vi "Check Properties Equal.vi"(8 "error in":errorcluster, 9 "Ignore Properties":string[](array[string]), 10 "BaseNodeType 2":refnum<k24>, 11 "BaseNodeType 1":refnum<k24>) -> (0 "error out":errorcluster, 1 "Equal?":bool, 2 "BaseNodeType 2":refnum<k24>, 3 "BaseNodeType 1":refnum<k24>, 4 "Inequality context":string)   [LabVIEW 2017, in "SLSC Switch Import Export Unit Tests.lvclass"]
uses:
  SLSC Switch Import Export Unit Tests.lvclass
  NationalInstruments.VeriStand.SystemStorage
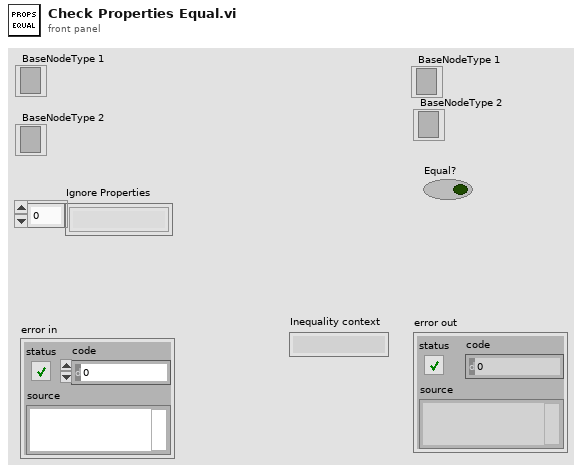
[diagram p1: front panel]
types:
  T1 = cluster{"ForceDownload":bool, "Path":string, "RTDestination":string, "Type":i32, "Version":string}
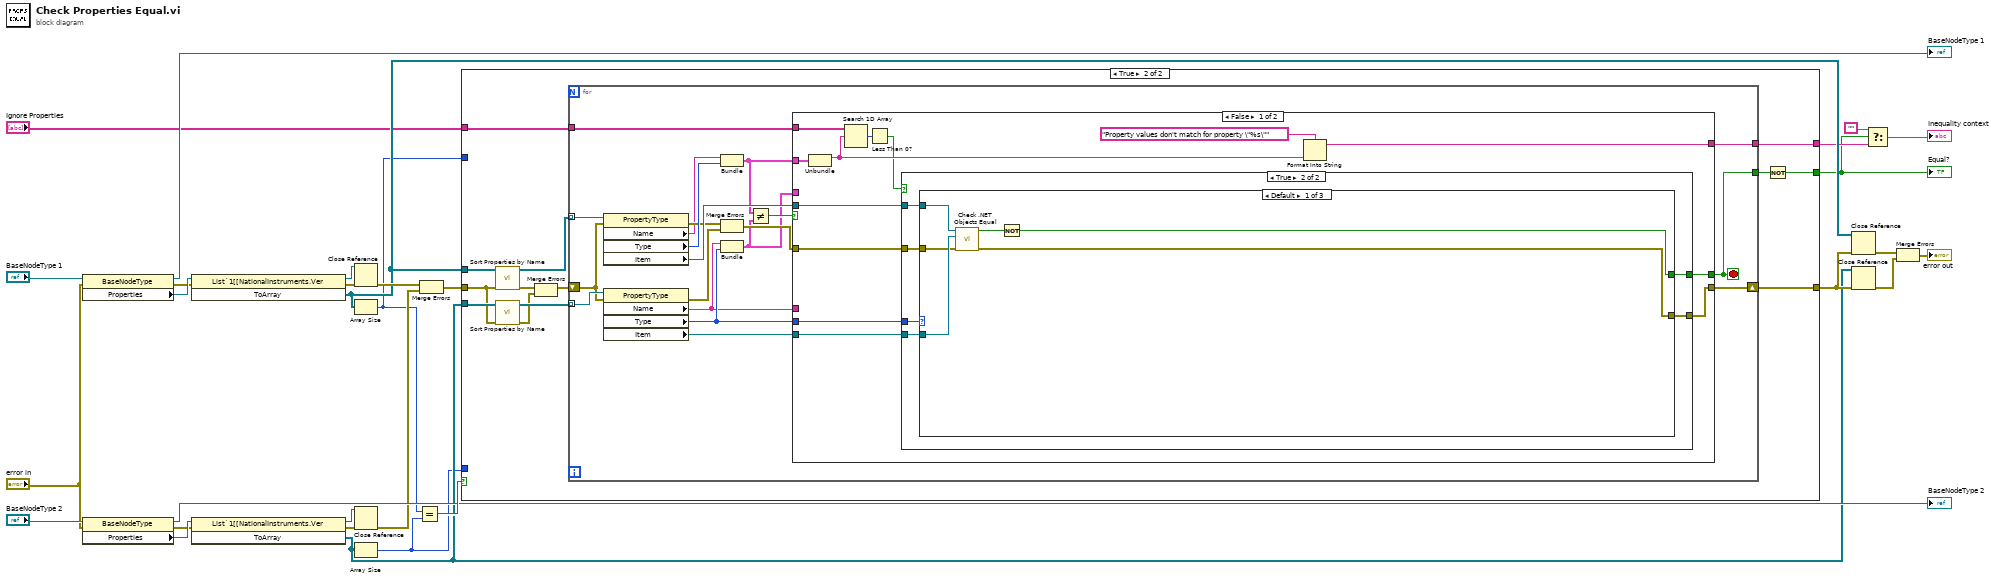
[diagram p0: block diagram]
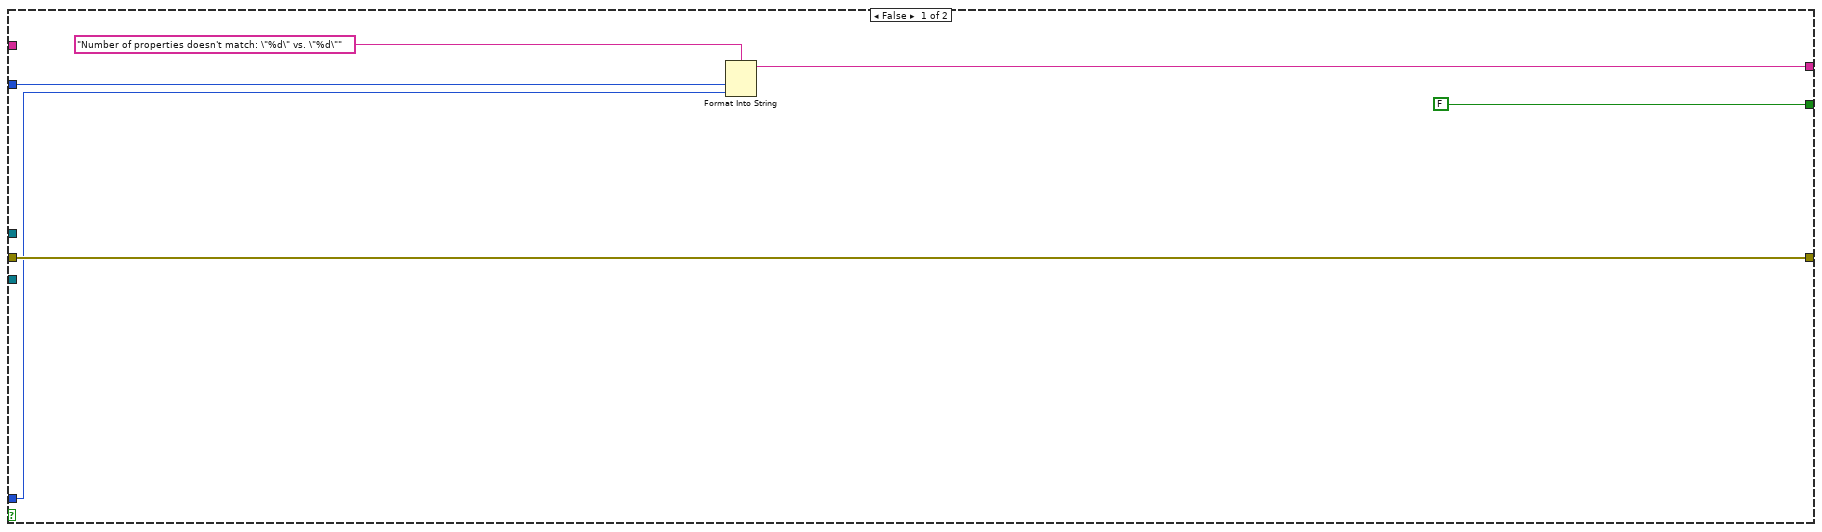
[diagram p2: hidden frame]
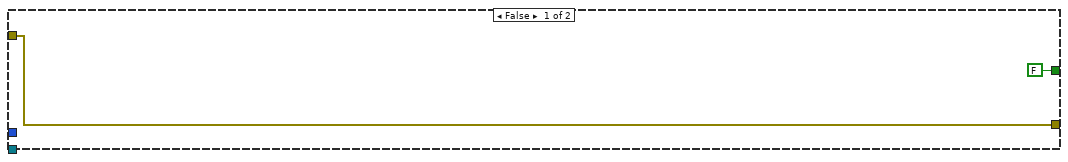
[diagram p3: hidden frame]
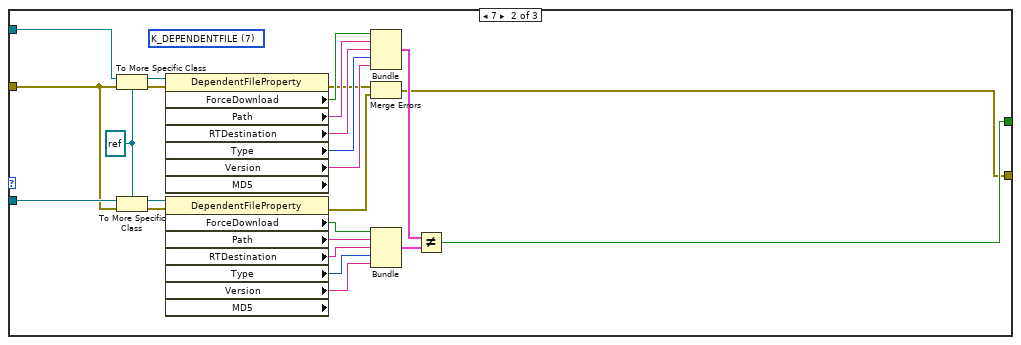
[diagram p4: hidden frame]
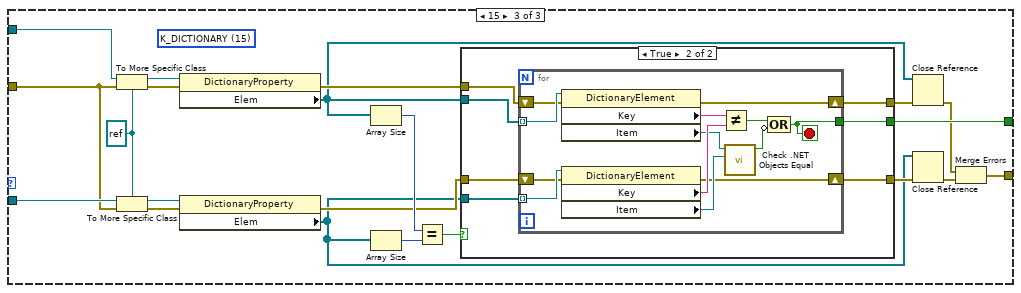
[diagram p5: hidden frame]
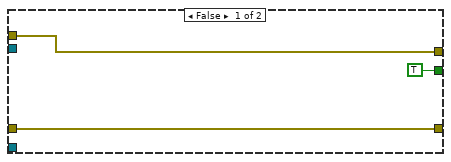
[diagram p6: hidden frame]
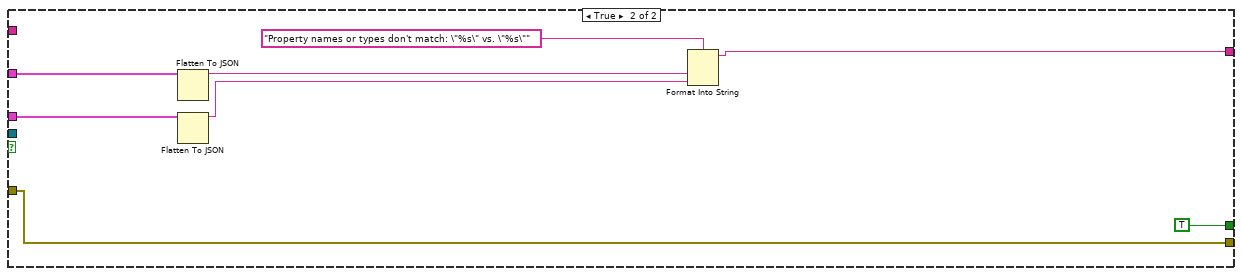
[diagram p7: hidden frame]
diagram:
  n1 = property class="BaseNodeType"(reference="BaseNodeType 1", error in="error in") -> (reference out=→"BaseNodeType 1":refnum<k24>, error out=w22:errorcluster, "Properties"=w29:refnum<k24>)
  n2 = property class="BaseNodeType"(reference="BaseNodeType 2", error in="error in") -> (reference out=→"BaseNodeType 2":refnum<k24>, error out=w21:errorcluster, "Properties"=w27:refnum<k24>)
  n3 = invoke class="List`1[[NationalInstruments.Ver" method="ToArray"(reference=w29, error in=w22) -> (reference out=w19:refnum<k24>, error out=w20:errorcluster, "ToArray"=w12:refnum<k24>[])  [unwired: 1 in]
  n4 = invoke class="List`1[[NationalInstruments.Ver" method="ToArray"(reference=w27, error in=w21) -> (reference out=w17:refnum<k24>, error out=w18:errorcluster, "ToArray"=w11:refnum<k24>[])  [unwired: 1 in]
  n5 = Close Reference(reference=w19, error in (no error)=w20) -> (error out=w16:errorcluster)
  n6 = Array Size(array=w12) -> (size(s)=w7:i32)
  n7 = Close Reference(reference=w17, error in (no error)=w18) -> (error out=w15:errorcluster)
  n8 = Array Size(array=w11) -> (size(s)=w6:i32)
  n9 = Equal?(x=w7, y=w6) -> (x = y?=w25:bool)
  n10 = Merge Errors(w16, w15) -> (w14:errorcluster)
  n11 = case shown="True" w25 {
    tunnel: w12 -> [_ w43]
    tunnel: w11 -> [_ w41]
    tunnel: [FALSE w49] -> w3
    tunnel: w14 -> [w35 w39]
    tunnel: [w35 w47] -> w13
    tunnel: w7 -> [w34 _]
    tunnel: w6 -> [w33 _]
    tunnel: [w32 w46] -> w4
    tunnel: "Ignore Properties" -> [_ w45]
    frame False {
      n12 = Format Into String(format string="Number of properties doesn't match: \"%d\" vs. \"%d\"", w34, w33) -> (resulting string=w32:string)  [unwired: 2 in, 1 out]
    }
    frame True {
      n13 = call "Sort Properties by Name.vi"("error in (no error)"=w39, "properties"=w43) -> ("error out"=w44:errorcluster, "sorted properties"=w42:refnum<k24>[])  [unwired: 8 in]
      n14 = call "Sort Properties by Name.vi"("error in (no error)"=w39, "properties"=w41) -> ("error out"=w37:errorcluster, "sorted properties"=w40:refnum<k24>[])  [unwired: 8 in]
      n15 = Merge Errors(w44, w37) -> (w38:errorcluster)
      n16 = for {
        tunnel: w42 -> [w68] mode=indexing
        tunnel: w40 -> [w67] mode=indexing
        tunnel: [w61] -> w48
        shift-right: [w56] -> w47
        shift-left: w38 -> [w60]
        tunnel: [w53] -> w46
        tunnel: w45 -> [w50]
        stop <- w61 stop-if-true
        n17 = property class="PropertyType"(reference=w68, error in=w60) -> (error out=w59:errorcluster, "Name"=w55:string, "Type"=w63:i32, "Item"=w65:refnum<k24>)  [unwired: 1 out]
        n18 = property class="PropertyType"(reference=w67, error in=w60) -> (error out=w58:errorcluster, "Name"=w54:string, "Type"=w64:i32, "Item"=w66:refnum<k24>)  [unwired: 1 out]
        n19 = Bundle("Name"=w55, "Type"=w63) -> (w52:cluster{"Name":string, "Type":i32})  [unwired: 1 in]
        n20 = Merge Errors(w59, w58) -> (w57:errorcluster)
        n21 = Bundle("Name"=w54, "Type"=w64) -> (w51:cluster{"Name":string, "Type":i32})  [unwired: 1 in]
        n22 = Not Equal?(x=w52, y=w51) -> (x != y?=w62:bool)
        n23 = case shown="False" w62 {
          tunnel: w66 -> [w80 _]
          tunnel: w65 -> [w79 _]
          tunnel: w64 -> [w78 _]
          tunnel: [w81 TRUE] -> w61
          tunnel: w57 -> [w77 w170]
          tunnel: [w76 w170] -> w56
          tunnel: w54 -> [_ _]
          tunnel: [w74 w168] -> w53
          tunnel: w52 -> [w73 w167]
          tunnel: w51 -> [_ w165]
          tunnel: w50 -> [w72 _]
          frame False {
            n24 = Unbundle(w73) -> ("Name"=w71:string)  [unwired: 1 out]
            n25 = Search 1D Array(1D array=w72, element=w71) -> (index of element=w70:i32)  [unwired: 1 in]
            n26 = Less Than 0?(x=w70) -> (x < 0?=w69:bool)
            n27 = case shown="True" w69 {
              tunnel: [FALSE w89] -> w81
              tunnel: w80 -> [_ w88]
              tunnel: w79 -> [_ w87]
              tunnel: w78 -> [_ w86]
              tunnel: w77 -> [w82 w85]
              tunnel: [w82 w84] -> w76
              frame False {
              }
              frame True {
                n28 = case shown="Default" w86 {
                  tunnel: w88 -> [w93 w116 w138]
                  tunnel: w87 -> [w94 w119 w139]
                  tunnel: [w95 w108 w133] -> w89
                  tunnel: w85 -> [w91 w99 w130]
                  tunnel: [w90 w96 w126] -> w84
                  frame Default {
                    n29 = call "Check .NET Objects Equal.vi"("error in"=w91, "object 2"=w93, "object 1"=w94) -> ("error out"=w90:errorcluster, "Equal?"=w92:bool)  [unwired: 7 in]
                    n30 = Not(x=w92) -> (.not. x?=w95:bool)
                  }
                  frame 7 {
                    (unwired) 7 items=["K_STRING", "K_BOOL", "K_I32", "K_U32", "K_DOUBLE", "K_U64", "K_VARIANT", "K_DEPENDENTFILE", "K_DEPENDENTNODE", "K_DATASOURCENODE", "K_U16", "K_DBLARR", "K_U32ARR", "K_I32ARR", "K_STRINGARR", "K_DICTIONARY", "K_DICTIONARYARR", "K_BINARYSTRING", "K_I16", "K_I64", "K_BOOLARR", "K_U64ARR", "K_U16ARR", "K_I64ARR", "K_I16ARR"] ("Type")
                    w115 = refnum<k24> refnum ("target class")
                    n31 = To More Specific Class(target class=w115, reference=w119, error in=w99) -> (specific class reference=w118:refnum<k24>, error out=w100:errorcluster)
                    n32 = To More Specific Class(target class=w115, reference=w116, error in=w99) -> (specific class reference=w117:refnum<k24>, error out=w101:errorcluster)
                    n33 = property class="DependentFileProperty" props=["ForceDownload", "Path", "RTDestination", "Type", "Version", "MD5"](reference=w118, error in=w100) -> (error out=w98:errorcluster, "ForceDownload"=w114:bool, "Path"=w113:string, "RTDestination"=w107:string, "Type"=w105:i32, "Version"=w103:string)  [unwired: 2 out]
                    n34 = property class="DependentFileProperty" props=["ForceDownload", "Path", "RTDestination", "Type", "Version", "MD5"](reference=w117, error in=w101) -> (error out=w97:errorcluster, "ForceDownload"=w112:bool, "Path"=w111:string, "RTDestination"=w106:string, "Type"=w104:i32, "Version"=w102:string)  [unwired: 2 out]
                    n35 = Bundle("ForceDownload"=w114, "Path"=w113, "RTDestination"=w107, "Type"=w105, "Version"=w103) -> (w110:T1)  [unwired: 1 in]
                    n36 = Merge Errors(w98, w97) -> (w96:errorcluster)
                    n37 = Bundle("ForceDownload"=w112, "Path"=w111, "RTDestination"=w106, "Type"=w104, "Version"=w102) -> (w109:T1)  [unwired: 1 in]
                    n38 = Not Equal?(x=w110, y=w109) -> (x != y?=w108:bool)
                  }
                  frame 15 {
                    w140 = refnum<k24> refnum ("target class")
                    (unwired) 15 items=["K_STRING", "K_BOOL", "K_I32", "K_U32", "K_DOUBLE", "K_U64", "K_VARIANT", "K_DEPENDENTFILE", "K_DEPENDENTNODE", "K_DATASOURCENODE", "K_U16", "K_DBLARR", "K_U32ARR", "K_I32ARR", "K_STRINGARR", "K_DICTIONARY", "K_DICTIONARYARR", "K_BINARYSTRING", "K_I16", "K_I64", "K_BOOLARR", "K_U64ARR", "K_U16ARR", "K_I64ARR", "K_I16ARR"] ("Type")
                    n39 = To More Specific Class(target class=w140, reference=w139, error in=w130) -> (specific class reference=w137:refnum<k24>, error out=w131:errorcluster)
                    n40 = To More Specific Class(target class=w140, reference=w138, error in=w130) -> (specific class reference=w132:refnum<k24>, error out=w129:errorcluster)
                    n41 = property class="DictionaryProperty"(reference=w137, error in=w131) -> (error out=w128:errorcluster, "Elem"=w121:refnum<k24>[])  [unwired: 1 out]
                    n42 = property class="DictionaryProperty"(reference=w132, error in=w129) -> (error out=w127:errorcluster, "Elem"=w120:refnum<k24>[])  [unwired: 1 out]
                    n43 = Array Size(array=w121) -> (size(s)=w135:i32)
                    n44 = Array Size(array=w120) -> (size(s)=w136:i32)
                    n45 = Equal?(x=w135, y=w136) -> (x = y?=w134:bool)
                    n46 = case shown="True" w134 {
                      tunnel: w121 -> [_ w150]
                      tunnel: w120 -> [_ w149]
                      tunnel: [TRUE w148] -> w133
                      tunnel: w128 -> [w142 w147]
                      tunnel: w127 -> [w141 w146]
                      tunnel: [w142 w145] -> w125
                      tunnel: [w141 w144] -> w124
                      frame False {
                      }
                      frame True {
                        n47 = for {
                          tunnel: w150 -> [w163] mode=indexing
                          tunnel: w149 -> [w162] mode=indexing
                          tunnel: [w159] -> w148
                          shift-right: [w151] -> w145
                          shift-left: w147 -> [w154]
                          shift-right: [w152] -> w144
                          shift-left: w146 -> [w153]
                          stop <- w159 stop-if-true
                          n48 = property class="DictionaryElement"(reference=w163, error in=w154) -> (error out=w151:errorcluster, "Key"=w161:string, "Item"=w156:refnum<k24>)  [unwired: 1 out]
                          n49 = property class="DictionaryElement"(reference=w162, error in=w153) -> (error out=w152:errorcluster, "Key"=w160:string, "Item"=w157:refnum<k24>)  [unwired: 1 out]
                          n50 = Not Equal?(x=w161, y=w160) -> (x != y?=w158:bool)
                          n51 = call "Check .NET Objects Equal.vi"("object 2"=w157, "object 1"=w156) -> ("Equal?"=w155:bool)  [unwired: 8 in, 1 out]
                          n52 = Compound Arithmetic op=OR(w158, invert w155) -> (w159:bool)
                        }
                      }
                    }
                    n53 = Close Reference(reference=w121, error in (no error)=w125) -> (error out=w123:errorcluster)
                    n54 = Close Reference(reference=w120, error in (no error)=w124) -> (error out=w122:errorcluster)
                    n55 = Merge Errors(w123, w122) -> (w126:errorcluster)
                  }
                }
              }
            }
            n56 = Format Into String(format string="Property values don't match for property \"%s\"", w71) -> (resulting string=w74:string)  [unwired: 2 in, 1 out]
          }
          frame True {
            n57 = Flatten To JSON(anything=w167) -> (JSON string=w166:string)  [unwired: 2 in, 1 out]
            n58 = Flatten To JSON(anything=w165) -> (JSON string=w164:string)  [unwired: 2 in, 1 out]
            n59 = Format Into String(format string="Property names or types don't match: \"%s\" vs. \"%s\"", w166, w164) -> (resulting string=w168:string)  [unwired: 2 in, 1 out]
          }
        }
      }
      n60 = Not(x=w48) -> (.not. x?=w49:bool)
    }
  }
  "Equal?" <- w3
  n61 = Close Reference(reference=w12, error in (no error)=w13) -> (error out=w10:errorcluster)
  n62 = Close Reference(reference=w11, error in (no error)=w13) -> (error out=w9:errorcluster)
  n63 = Select(t="", s=w3, f=w4) -> (s? t:f=→"Inequality context":string)
  n64 = Merge Errors(w10, w9) -> (→"error out":errorcluster)
